vi "ode fcn template.vi"(6 "params":dbl[](array[numeric]), 9 "F":dbl[](array[numeric]), 11 "y":dbl[](array[numeric])) -> (3 "dydt":dbl[](array[numeric]))   [LabVIEW 2010, in "common.lvlib"]
uses:
  common-lvlib/common.lvlib
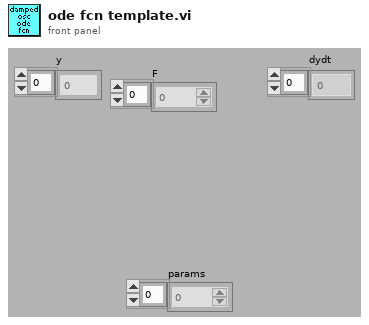
[diagram p1: front panel]
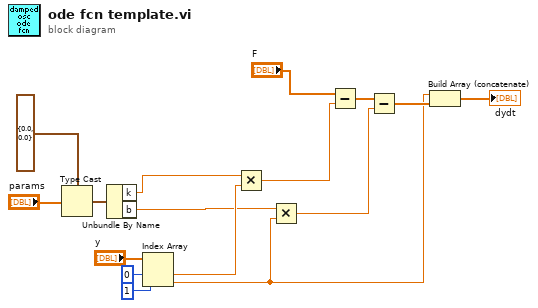
[diagram p0: block diagram]
diagram:
  n1 = Type Cast(type=cluster{"k":dbl, "b":dbl} {"k"=0.0, "b"=0.0}, x="params") -> (*(type *) &x=w3:cluster{"k":dbl, "b":dbl})
  n2 = Unbundle By Name(w3) -> ("k"=w2:dbl, "b"=w1:dbl)
  n3 = Index Array(array="y", index #1=0 ("index"), index #2=1 ("index")) -> (element #1=w13:dbl, element #2=w8:dbl)
  n4 = Multiply(x=w2, y=w13) -> (x*y=w12:dbl)
  n5 = Multiply(x=w1, y=w8) -> (x*y=w10:dbl)
  n6 = Subtract(x="F", y=w12) -> (x-y=w11:dbl[])
  n7 = Subtract(x=w11, y=w10) -> (x-y=w9:dbl[])
  n8 = Build Array (concatenate)(w8, w9) -> (→"dydt":dbl[])
